vi "GetIntegrationRate.vi"(8 "Error In":errorcluster, 10 "Channel (1 or 2)":u8 min=1 max=2 step=1, 11 "Keithley 6482 In":refnum<visa-resource-name>) -> (0 "Error Out":errorcluster, 2 "Integration Rate":dbl, 3 "Keithley 6482 Out":refnum<visa-resource-name>)   [LabVIEW 2009, in "Keithley-6482-Visa.lvlib"]
uses:
  <instrlib>/Keithley-6482-Visa9.0/Keithley-6482-Visa.lvlib
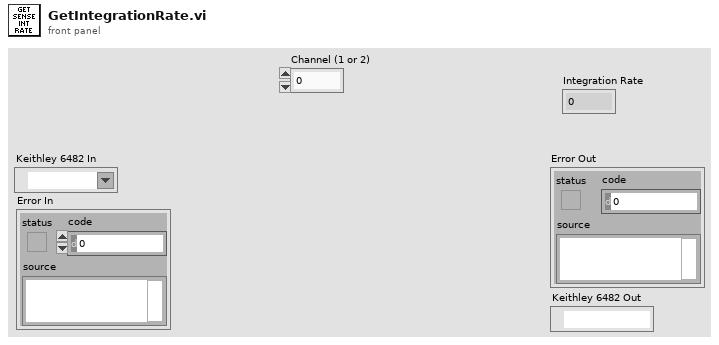
[diagram p1: front panel]
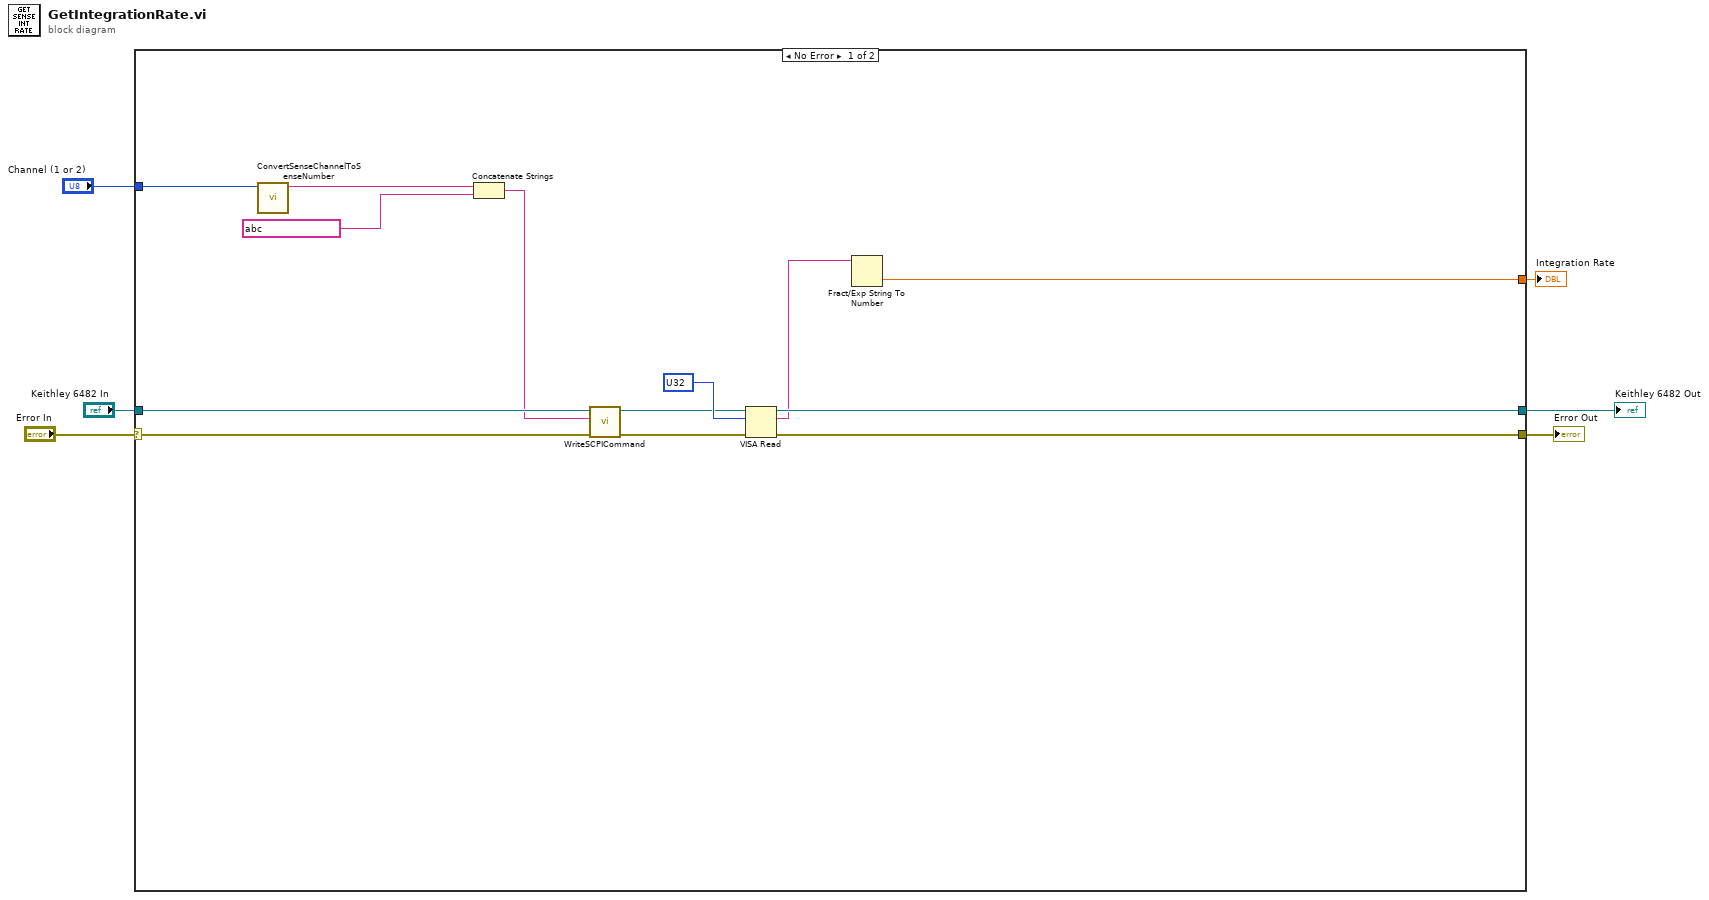
[diagram p0: block diagram]
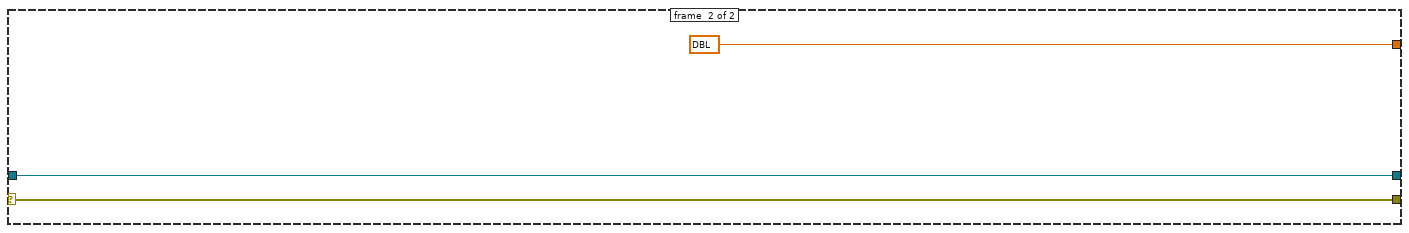
[diagram p2: hidden frame]
diagram:
  n1 = case shown="No Error" "Error In" {
    selector: "Error In" -> [w14 w21]
    tunnel: "Keithley 6482 In" -> [w13 w22]
    tunnel: [w19 w21] -> w4
    tunnel: [w18 w22] -> w3
    tunnel: "Channel (1 or 2)" -> [w12 _]
    tunnel: [w7 dbl ?] -> w1
    frame #0 {
      n2 = call <instrlib>:"ConvertSenseChannelToSenseNumber.vi"("Channel (1 or 2)"=w12) -> ("Sense Number"=w11:string)  [unwired: 10 in]
      n3 = Concatenate Strings(w11, string ? ("string")) -> (w9:string)
      n4 = call <instrlib>:"WriteSCPICommand.vi"("Error In"=w14, "SCPI Command"=w9, "Keithley 6482 In"=w13) -> ("Error Out"=w15:errorcluster, "Keithley 6482 Out"=w16:refnum<visa-resource-name>)  [unwired: 7 in]
      n5 = VISA Read(VISA resource name=w16, byte count=u32 ?, error in (no error)=w15) -> (VISA resource name out=w18:refnum<visa-resource-name>, read buffer=w8:string, error out=w19:errorcluster)  [unwired: 1 out]
      n6 = Fract/Exp String To Number(string=w8) -> (number=w7:dbl)  [unwired: 3 in, 1 out]
    }
    frame #1 {
    }
  }
  "Error Out" <- w4
  "Keithley 6482 Out" <- w3
  "Integration Rate" <- w1
